vi "Send Receive Queue.vi"(4 "timeout in ms (-1)":i32, 6 "Write (T)":bool, 7 "Queue":string, 8 "error in (no error)":errorcluster, 11 "Data In":variant) -> (0 "error out":errorcluster, 3 "Data Out":variant)   [LabVIEW 2017]
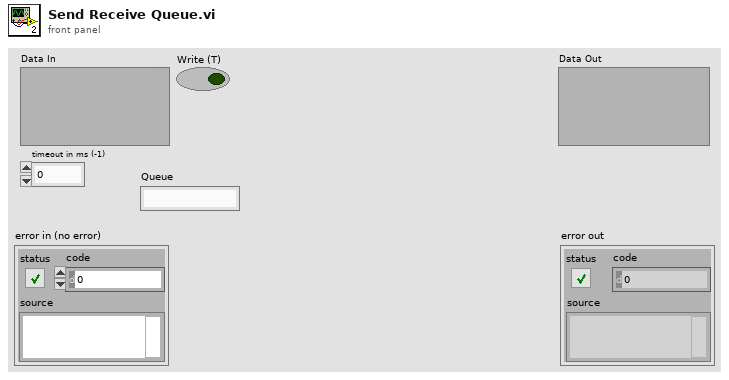
[diagram p1: front panel]
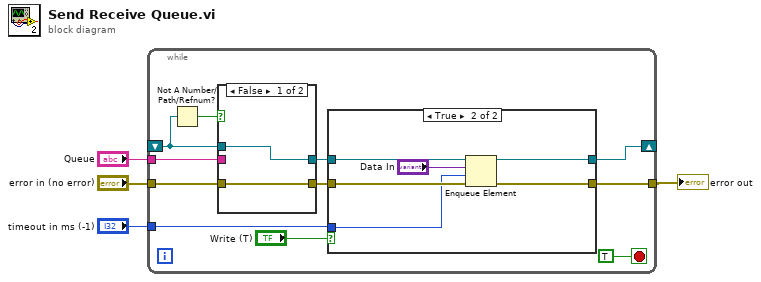
[diagram p0: block diagram]
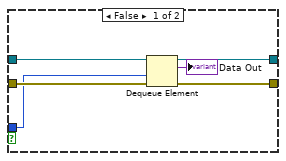
[diagram p2: hidden frame]
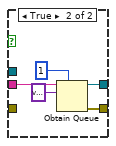
[diagram p3: hidden frame]
diagram:
  n1 = while {
    tunnel: "Queue" -> [w15]
    shift-right: [w11] -> _
    shift-left: _ -> [w12]
    tunnel: [w9] -> w1
    tunnel: "timeout in ms (-1)" -> [w8]
    tunnel: "error in (no error)" -> [w7]
    stop <- TRUE stop-if-true
    n2 = Not A Number/Path/Refnum?(number/path/refnum=w12) -> (NaN/Path/Refnum?=w13:bool)
    n3 = case shown="False" w13 {
      tunnel: w15 -> [_ w34]
      tunnel: [w29 w32] -> w14
      tunnel: w12 -> [w29 _]
      tunnel: [w28 w30] -> w10
      tunnel: w7 -> [w28 _]
      frame False {
      }
      frame True {
        n4 = Obtain Queue(max queue size (-1, unlimited)=1, name (unnamed)=w34, element data type=variant) -> (queue out=w32:refnum<queue>, error out=w30:errorcluster)  [unwired: 2 in, 1 out]
      }
    }
    n5 = case shown="True" "Write (T)" {
      tunnel: w14 -> [w21 w27]
      tunnel: [w20 w26] -> w11
      tunnel: w10 -> [w19 w25]
      tunnel: [w18 w24] -> w9
      tunnel: w8 -> [w16 w22]
      frame False {
        n6 = Dequeue Element(queue=w21, timeout in ms (-1)=w16, error in (no error)=w19) -> (queue out=w20:refnum<queue>, element=→"Data Out":variant, error out=w18:errorcluster)  [unwired: 1 out]
      }
      frame True {
        n7 = Enqueue Element(queue=w27, element="Data In", timeout in ms (-1)=w22, error in (no error)=w25) -> (queue out=w26:refnum<queue>, error out=w24:errorcluster)  [unwired: 1 out]
      }
    }
  }
  "error out" <- w1
